vi "Get Wheel Parameter by Name as String.vi"(8 "error in (no error)":errorcluster, 10 "parameter name":string, 11 "wheel in":refnum<class "NI_Robotics_Caster Wheel.lvclass">) -> (0 "error out":errorcluster, 1 "found?":bool, 2 "parameter value":string, 3 "wheel out":refnum<class "NI_Robotics_Caster Wheel.lvclass">)   [LabVIEW 2017, in "NI_Robotics_Caster Wheel.lvclass"]
uses:
  <vilib>/robotics/Steering/Caster Wheel/NI_Robotics_Caster Wheel.lvclass
  <vilib>/robotics/Steering/Caster Wheel/NI_Robotics_Caster Wheel.lvclass/NI_Robotics_Caster Wheel.ctl
  <vilib>/robotics/Actuation/Motor Communication/NI_Robotics_Motor Communication.lvclass/NI_Robotics_Motor Communication.ctl
  <vilib>/robotics/Steering/Wheel/NI_Robotics_Wheel.lvclass
  <vilib>/robotics/Actuation/Motor Communication/NI_Robotics_Motor Communication.lvclass
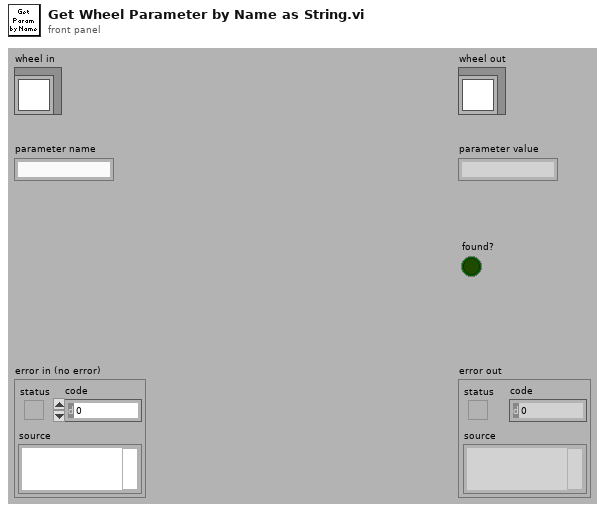
[diagram p1: front panel]
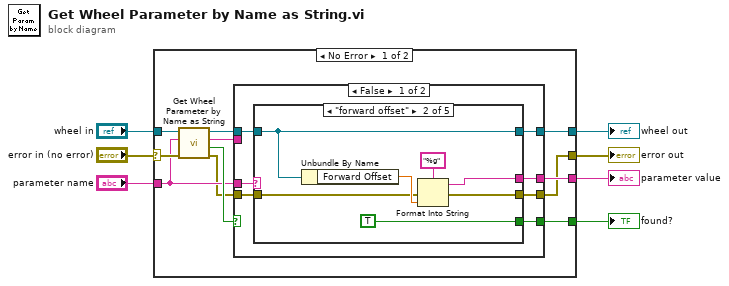
[diagram p0: block diagram]
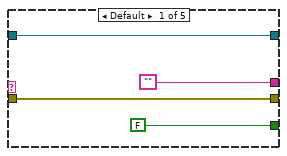
[diagram p2: hidden frame]
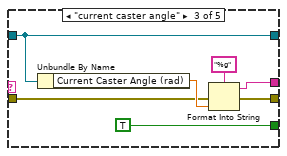
[diagram p3: hidden frame]
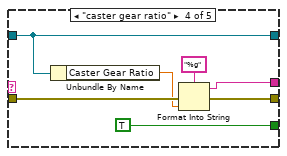
[diagram p4: hidden frame]
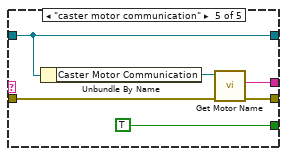
[diagram p5: hidden frame]
diagram:
  n1 = case shown="No Error" "error in (no error)" {
    selector: "error in (no error)" -> [w17 w61]
    tunnel: [w8 w61] -> w3
    tunnel: [w11 _] -> w2
    tunnel: [w12 _] -> w1
    tunnel: [w13 w62] -> w4
    tunnel: "parameter name" -> [w10 _]
    tunnel: "wheel in" -> [w18 w62]
    frame No Error {
      n2 = call-parent "Get Wheel Parameter by Name as String.vi"("error in (no error)"=w17, "parameter name"=w10, "wheel in"=w18) -> ("error out"=w9:errorcluster, "found?"=w16:bool, "parameter value"=w15:string, "wheel out"=w14:refnum<class "NI_Robotics_Caster Wheel.lvclass">)  [unwired: 5 in]
      n3 = case shown="False" w16 {
        selector: w16 -> [_ w58]
        tunnel: w15 -> [_ w59]
        tunnel: w14 -> [w24 w60]
        tunnel: [w23 w60] -> w13
        tunnel: [w22 w59] -> w12
        tunnel: [w21 w58] -> w11
        tunnel: w10 -> [w25 _]
        tunnel: w9 -> [w20 w57]
        tunnel: [w19 w57] -> w8
        frame False {
          n4 = case shown="\"forward offset\"" w25 {
            tunnel: w24 -> [w29 w36 w42 w50 w56]
            tunnel: [w29 w36 w42 w50 w56] -> w23
            tunnel: ["" ("parameter value") w32 w37 w44 w53] -> w22
            tunnel: [FALSE TRUE TRUE TRUE TRUE] -> w21
            tunnel: w20 -> [w26 w31 w39 w47 w51]
            tunnel: [w26 w30 w38 w45 w52] -> w19
            frame Default {
            }
            frame "forward offset" {
              n5 = Unbundle By Name(w36) -> ("Forward Offset"=w33:dbl)
              n6 = Format Into String(format string="%g", error in=w31, w33) -> (resulting string=w32:string, error out=w30:errorcluster)  [unwired: 1 in]
            }
            frame "current caster angle" {
              n7 = Unbundle By Name(w42) -> ("Current Caster Angle (rad)"=w40:dbl)
              n8 = Format Into String(format string="%g", error in=w39, w40) -> (resulting string=w37:string, error out=w38:errorcluster)  [unwired: 1 in]
            }
            frame "caster gear ratio" {
              n9 = Unbundle By Name(w50) -> ("Caster Gear Ratio"=w46:dbl)
              n10 = Format Into String(format string="%g", error in=w47, w46) -> (resulting string=w44:string, error out=w45:errorcluster)  [unwired: 1 in]
            }
            frame "caster motor communication" {
              n11 = Unbundle By Name(w56) -> ("Caster Motor Communication"=w54:refnum<class "NI_Robotics_Motor Communication.lvclass">)
              n12 = call <vilib>:"Get Motor Name.vi"("error in (no error)"=w51, "motor communication in"=w54) -> ("error out"=w52:errorcluster, "motor name"=w53:string)  [unwired: 7 in, 1 out]
            }
          }
        }
        frame True {
        }
      }
    }
    frame Error {
    }
  }
  "error out" <- w3
  "wheel out" <- w4
  "found?" <- w2
  "parameter value" <- w1
